vi "Launch Asynchronous VI.vi"(8 "error in (no error)":errorcluster, 10 "VI path":path) -> (0 "error out":errorcluster)   [LabVIEW 2011]
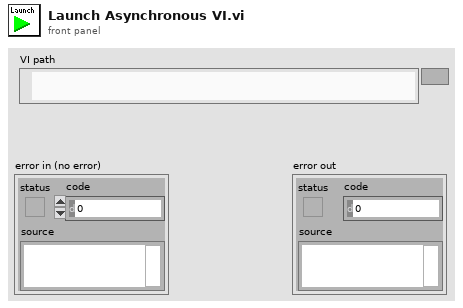
[diagram p1: front panel]
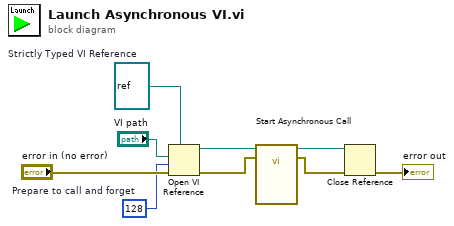
[diagram p0: block diagram]
diagram:
  w6 = 128  # Prepare to call and forget
  w8 = refnum<vi> refnum  # Strictly Typed VI Reference
  n1 = Open VI Reference(type specifier VI Refnum (for type only)=w8, vi path="VI path", options=w6, error in (no error)="error in (no error)") -> (vi reference=w2:refnum<vi>, error out=w1:errorcluster)  [unwired: 2 in]
  n2 = call-by-ref "Start Asynchronous Call"(reference=w2, error in=w1) -> (reference out=w4:refnum<vi>, error out=w5:errorcluster)  [unwired: 11 in, 1 out]
  n3 = Close Reference(reference=w4, error in (no error)=w5) -> (error out=→"error out":errorcluster)
